vi "RegisterTrend.vi"(8 "error in":errorcluster, 10 "RegisterTrend":T2, 11 "config":T1) -> (0 "error out":errorcluster, 3 "config out":T1)   [LabVIEW 2017, in "EmsaDataEventCreator.lvlib"]
uses:
  <vilib>/addons/InsightCM/Devices/Shared/Emsa/EmsaDataEventCreator/EmsaDataEventCreator.lvlib
  <vilib>/addons/InsightCM/Devices/Shared/Common/DataEventCreator/controls/RegisterTrendPoints.ctl
  <vilib>/addons/InsightCM/Devices/Shared/Common/DataEventCreator/controls/Registry_Trend.ctl
  <vilib>/addons/InsightCM/Devices/Shared/Emsa/EmsaDataEventCreator/controls/config.ctl
  <vilib>/addons/InsightCM/Devices/Shared/Emsa/EmsaDataEventCreator/controls/Registry.ctl
  <vilib>/addons/InsightCM/Devices/Shared/Emsa/EmsaDataEventCreator/controls/Registry_Sweep.ctl
  <vilib>/addons/InsightCM/Devices/Shared/Common/DataEvent/controls/DataSetType.ctl
  <vilib>/addons/InsightCM/MessageBus/Base/controls/KeyValuePair.ctl
  <vilib>/addons/InsightCM/Devices/Shared/Common/DataEventCreator/DataEventCreator.lvlib
  <vilib>/addons/InsightCM/Devices/Shared/Common/DataEvent/DataEvent.lvlib
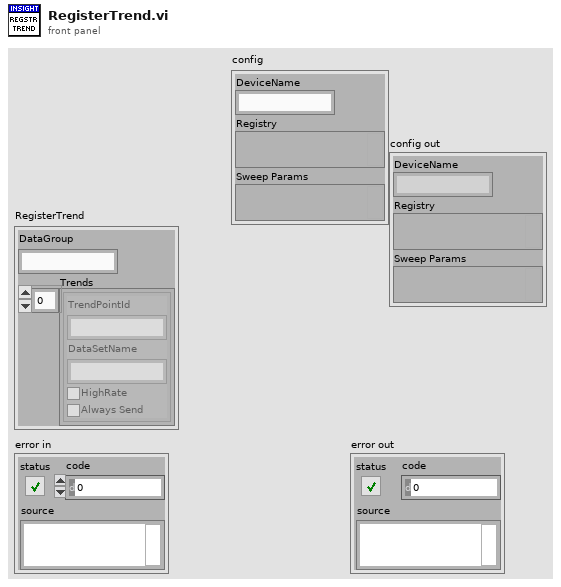
[diagram p1: front panel]
types:
  T1 = typedef "EmsaDataEventCreator.lvlib/config.ctl" = cluster{"DeviceName":string, "Registry":variant, "Sweep Params":variant}
  T2 = typedef "DataEventCreator.lvlib/RegisterTrendPoints.ctl" = cluster{"DataGroup":string, "Trends":T3[]}
  T3 = typedef "DataEventCreator.lvlib/Registry_Trend.ctl" = cluster{"TrendPointId":string, "DataSetName":string, "HighRate":bool, "Always Send":bool}
  T4 = typedef "EmsaDataEventCreator.lvlib/Registry.ctl" = cluster{"Sweep Registry":T5[], "Trend Points":T3[], "AssetNodeMap":variant}
  T5 = typedef "EmsaDataEventCreator.lvlib/Registry_Sweep.ctl" = cluster{"Name":string, "DataSetType":T6, "Properties":T7[]}
  T6 = typedef "DataEvent.lvlib/DataSetType.ctl" = enum16{"Waveform", "SpeedProfile", "ThermalImage", "EmsaSweep"}
  T7 = typedef "KeyValuePair.ctl" = cluster{"Key":string, "Value":string}
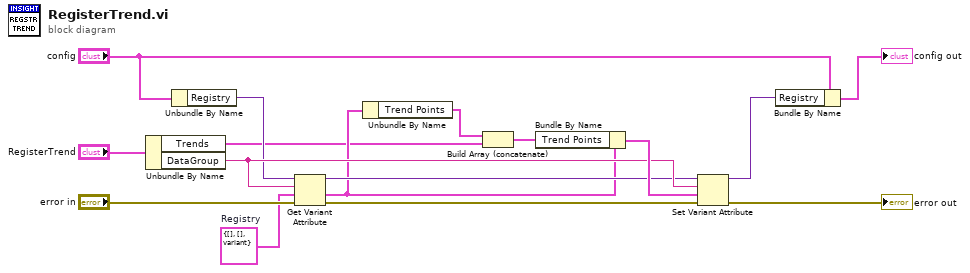
[diagram p0: block diagram]
diagram:
  w1 = T4 {"Sweep Registry"=[], "Trend Points"=[], "AssetNodeMap"=variant}  # Registry
  n1 = Unbundle By Name("RegisterTrend") -> ("Trends"=w6:T3[], "DataGroup"=w14:string)
  n2 = Unbundle By Name("config") -> ("Registry"=w12:variant)
  n3 = Get Variant Attribute(Variant=w12, name=w14, default value (empty Variant)=w1, error in="error in") -> (duplicate Variant=w13:variant, value=w8:T4, error out=w16:errorcluster)  [unwired: 1 out]
  n4 = Unbundle By Name(w8) -> ("Trend Points"=w7:T3[])
  n5 = Build Array (concatenate)(w7, w6) -> (w5:T3[])
  n6 = Bundle By Name(cluster=w8, "Trend Points"=w5) -> (w15:T4)
  n7 = Set Variant Attribute(Variant=w13, name=w14, value=w15, error in=w16) -> (Variant out=w11:variant, error out=→"error out":errorcluster)  [unwired: 1 out]
  n8 = Bundle By Name(cluster="config", "Registry"=w11) -> (→"config out":T1)
